vi "MC Test Data Path.vi"(7 "Append Name":string, 9 "Save Test Data":bool, 10 "State":enum16{"Initialise", "Write", "Read"}(ring)) -> (0 "error out":errorcluster, 1 "Save Test Data":bool, 3 "Test GraphData Path":path)   [LabVIEW 2020]
uses:
  Typedefs/Read Write Enum.ctl
  Global Variables/gl_UI Ctrl Refs.vi
  Global Variables/General Globals.vi
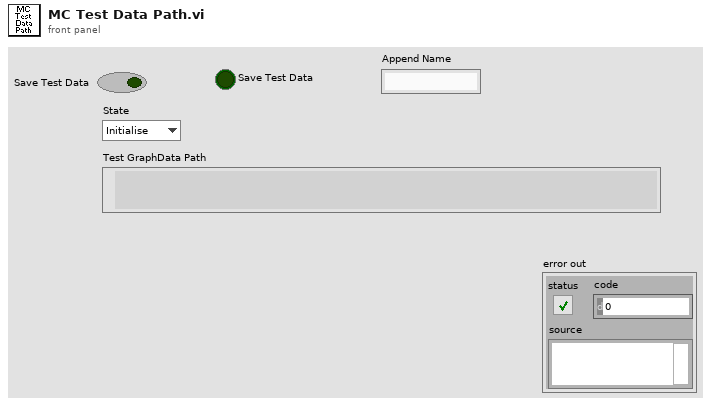
[diagram p1: front panel]
types:
  T1 = typedef "Read Write Enum.ctl" = enum16{"Read", "Write"}
  T2 = typedef "UI ctrl refs cluster.ctl" = cluster{"Top level VI path":path, "Top level VI ref":refnum<vi>, "User menu ref":refnum<k9>, "Sub Panel control":refnum<vi>, "Imaging Param Tab":refnum<vi>, "Occurrence-Start drivers":refnum<k4>, "Occurrence-Speed logging initialised":refnum<k4>, "Occurrence-XYZ stage initialised":refnum<k4>, "Exit button":refnum<vi>, "Status ind":refnum<vi>, "Set as origin":refnum<vi>, "Speed Logging":refnum<vi>, "Time Lapse":refnum<vi>, "Live Imaging":refnum<vi>, "AOL Z Stack":refnum<vi>, "Motor Z Stack":refnum<vi>, "Funct Acq button":refnum<vi>, "Hard Shutter":refnum<vi>, "Virtual Shutter":refnum<vi>, "Laser Power":refnum<vi>, "AOL Mode":refnum<vi>, "Frame Size":refnum<vi>, "Field of View":refnum<vi>, "Dwell Time":refnum<vi>, "Zoom":refnum<vi>, "AOL Z":refnum<vi>, "Objective":refnum<vi>, "Axis":refnum<vi>, "Paths & Names":refnum<vi>, "Experiment folder path (ind.)":refnum<vi>, "Last State (Ind.)":refnum<vi>, "Averages":refnum<vi>, "Angle (degrees)":refnum<vi>, "X centre":refnum<vi>, "Y centre":refnum<vi>, "Plane Mode":refnum<vi>, "# Planes":refnum<vi>, "Z Start":refnum<vi>, "Z Stop":refnum<vi>, "Z Step":refnum<vi>, "PMT 1":refnum<vi>, "PMT 2":refnum<vi>, "Stage XYZ Position":refnum<vi>, "Pockels@Z Start":refnum<vi>, "Pockels@Z Stop":refnum<vi>, "Obtain Z Start":refnum<vi>, "Obtain Z Stop":refnum<vi>, "Live stim.trig.period":refnum<vi>, "Live stim.trig.enable":refnum<vi>, "Movement Correction":refnum<vi>, "Load Reference Image":refnum<vi>, "XY Stage Move":refnum<vi>, "MovCor Cluster":refnum<vi>, "RefDAQParam":refnum<vi>, "Funct. Acq. Pockels Modulation":refnum<vi>, "Ref Laser Power":refnum<vi>, "Enable Video Recording":refnum<vi>, "Video Record-Live Imaging":refnum<vi>, "Video Record-Funct acq":refnum<vi>, "Reference Source":refnum<vi>, "AOL Z-stack Chirps Ready (ind)":refnum<vi>, "Target time between mov.cor. ref triggers (ms)":refnum<vi>, "Funct. Acq. Ref frame save":refnum<vi>, "Tracking button":refnum<vi>, "Show ref plots window":refnum<vi>, "Center freq ind (nm)":refnum<vi>, "Pickup mode (ind)":refnum<vi>, "Logging queue (ind)":refnum<vi>, "Back aperture power (ind.)":refnum<vi>, "Power after objective (ind.)":refnum<vi>, "Switch user":refnum<vi>, "Ls1 Conn. Status":refnum<vi>, "Ls1Tuning Status":refnum<vi>, "Ls1 Faults":refnum<vi>, "Ls1 Connection":refnum<vi>, "Ls1 Mode":refnum<vi>, "Ls1 POWER [mW]":refnum<vi>, "Ls1Shutter":refnum<vi>, "Ls1 Wavelength":refnum<vi>, "Ls1 Note":refnum<vi>, "Ls1 Confirm Wav":refnum<vi>, "Ls1 PreChrp Prism1":refnum<vi>, "Ls1 PreChrp Prism2":refnum<vi>, "Ls1 wav top Ind":refnum<vi>, "Ls1 power top Ind":refnum<vi>, "Ls1 Pump peak Hold":refnum<vi>, "Ls1 Status Ind":refnum<vi>, "Ls1 wav cancel":refnum<vi>, "Experiment Type":refnum<vi>, "Biology Information":refnum<vi>, "Camera recording status":refnum<vi>}
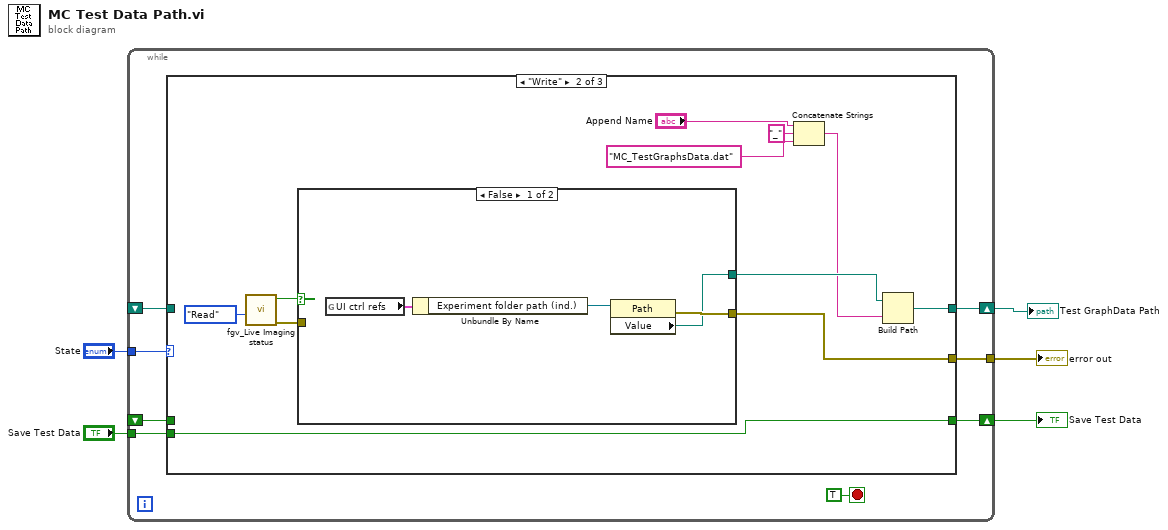
[diagram p0: block diagram]
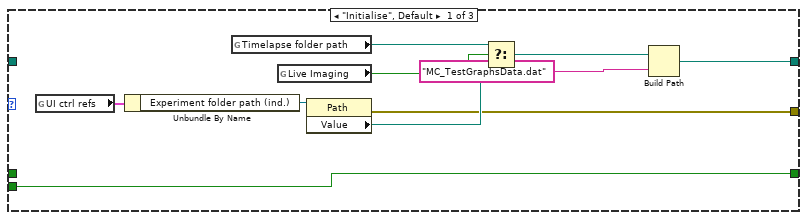
[diagram p2: hidden frame]
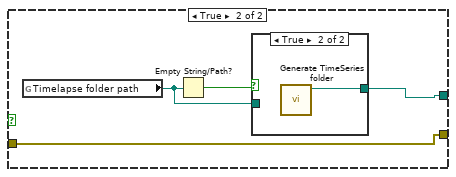
[diagram p3: hidden frame]
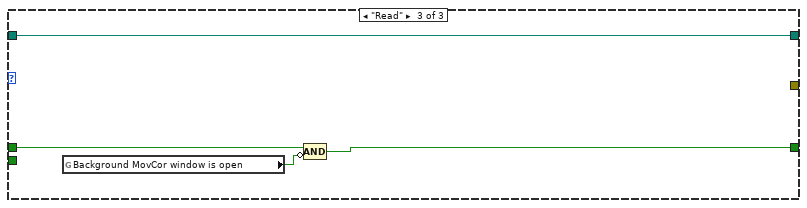
[diagram p5: hidden frame]
diagram:
  n1 = while {
    tunnel: "State" -> [w12]
    shift-right: [w10] -> w3
    shift-left: _ -> [w9]
    shift-right: [w11] -> w4
    shift-left: _ -> [w8]
    tunnel: "Save Test Data" -> [w7]
    tunnel: [w6] -> w1
    stop <- TRUE stop-if-true
    n2 = case shown="\"Write\"" w12 {
      tunnel: [w15 w33 w46] -> w11
      tunnel: [w16 w34 w48] -> w10
      tunnel: w9 -> [_ _ w48]
      tunnel: w8 -> [_ _ w45]
      tunnel: w7 -> [w15 w33 _]
      tunnel: [w14 w31 _] -> w6
      frame "Initialise", Default {
        n3 = global read "gl_UI Ctrl Refs.vi" "UI ctrl refs"() -> (w22:T2)
        n4 = Unbundle By Name(w22) -> ("Experiment folder path (ind.)"=w21:refnum<vi>)
        n5 = global read "General Globals.vi" "Timelapse folder path"() -> (w19:path)
        n6 = global read "General Globals.vi" "Live Imaging"() -> (w20:bool)
        n7 = property class="Path"(reference=w21) -> (error out=w14:errorcluster, "Value"=w18:path)  [unwired: 1 in, 1 out]
        n8 = Select(t=w19, s=w20, f=w18) -> (s? t:f=w17:path)
        n9 = Build Path(base path=w17, name or relative path="MC_TestGraphsData.dat") -> (appended path=w16:path)
      }
      frame "Write" {
        n10 = call "fgv_Live Imaging status.vi"("Function"=Read_Write_Enum."Read") -> ("error out"=w28:errorcluster, "Live Imaging?"=w30:bool)  [unwired: 9 in]
        n11 = case shown="False" w30 {
          tunnel: [w38 w42] -> w31
          tunnel: [w37 w41] -> w29
          tunnel: w28 -> [_ w42]
          frame False {
            n12 = global read "gl_UI Ctrl Refs.vi" "UI ctrl refs"() -> (w36:T2)
            n13 = Unbundle By Name(w36) -> ("Experiment folder path (ind.)"=w35:refnum<vi>)
            n14 = property class="Path"(reference=w35) -> (error out=w38:errorcluster, "Value"=w37:path)  [unwired: 1 in, 1 out]
          }
          frame True {
            n15 = global read "General Globals.vi" "Timelapse folder path"() -> (w39:path)
            n16 = Empty String/Path?(string/path=w39) -> (empty?=w40:bool)
            n17 = case shown="True" w40 {
              tunnel: [w43 w44] -> w41
              tunnel: w39 -> [w43 _]
              frame False {
              }
              frame True {
                n18 = call "Generate TimeSeries folder.vi"() -> ("Timelapse folder path"=w44:path)  [unwired: 10 in, 1 out]
              }
            }
          }
        }
        n19 = Concatenate Strings("Append Name", "_" ("string"), "MC_TestGraphsData.dat" ("name or relative path")) -> (w26:string)
        n20 = Build Path(base path=w29, name or relative path=w26) -> (appended path=w34:path)
      }
      frame "Read" {
        n21 = global read "General Globals.vi" "Background MovCor window is open"() -> (w47:bool)
        n22 = Compound Arithmetic op=AND(w45, invert w47) -> (w46:bool)
      }
    }
  }
  "Test GraphData Path" <- w3
  "Save Test Data" <- w4
  "error out" <- w1
